vi "Node.Settings.vi"(6 "Action":enum8{"Get", "Set"}(ring), 8 "error in (no error)":errorcluster, 10 "Node.Settings":T1 {"Name" format="%.0x"}, 11 "Item Ref in":T2 format="%.0x") -> (0 "error out":errorcluster, 2 "Node.Settings":T1 {"Name" format="%.0x"}, 3 "Item Ref out":T2 format="%.0x")   [LabVIEW 2023, in "J1939 Addon Shared.lvlib"]
uses:
  J1939 Addon Shared.lvlib
  <vilib>/NI VeriStand/Custom Device API/Custom Device Item Ref.ctl
  Types/Monitor Settings.ctl
  Constants.vi
  <vilib>/NI/NI VeriStand Advanced SysDef API/_SubVIs/SysDef.Property.Set.U32.vi
  <vilib>/NI/NI VeriStand Advanced SysDef API/_SubVIs/SysDef.Property.Set.String.vi
  <vilib>/NI/NI VeriStand Advanced SysDef API/_SubVIs/SysDef.Property.Set.Boolean.vi
  <vilib>/NI VeriStand/Custom Device API/Get Item Property (U32).vi
  <vilib>/NI VeriStand/Custom Device API/Get Item Property (String).vi
  <vilib>/NI VeriStand/Custom Device API/Get Item Property (Boolean).vi
  <vilib>/NI VeriStand/Custom Device API/Custom Device API.lvlib
  <vilib>/NI/NI VeriStand Advanced SysDef API/SysDef API/Advanced System Definition.lvlib
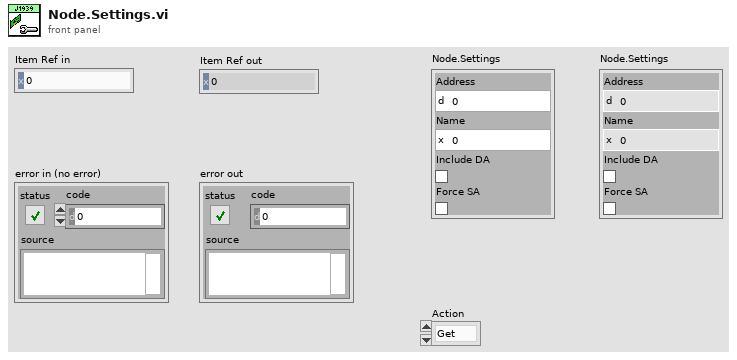
[diagram p1: front panel]
types:
  T1 = typedef "J1939 Addon Shared.lvlib/Monitor Settings.ctl" = cluster{"Address":u8, "Name":u64, "Include DA":bool, "Force SA":bool}
  T2 = typedef "Custom Device API.lvlib/Custom Device Item Ref.ctl" = u64
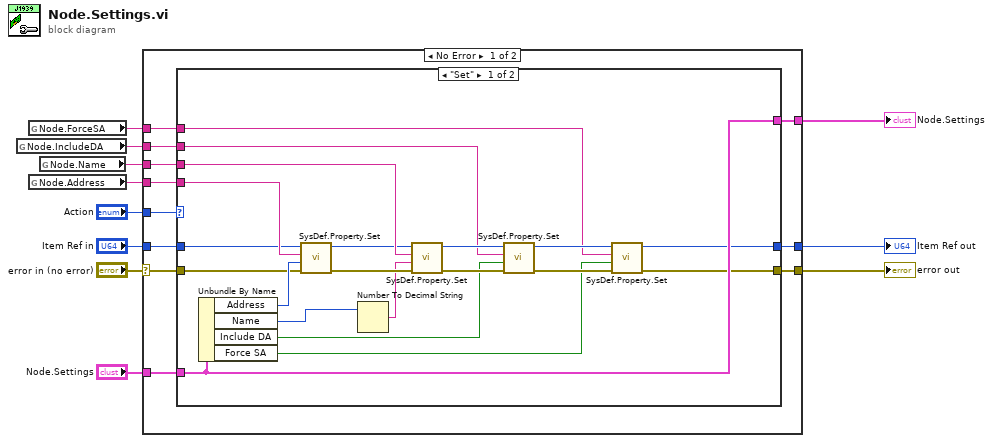
[diagram p0: block diagram]
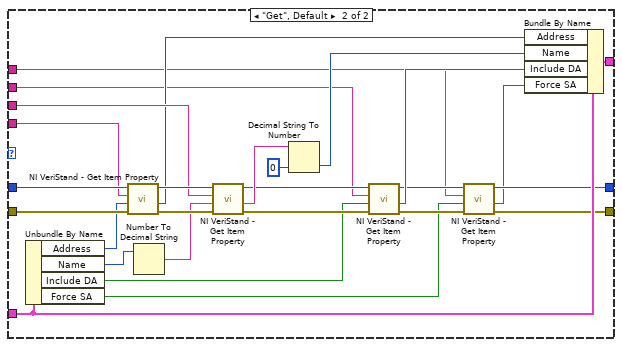
[diagram p2: hidden frame]
diagram:
  n1 = global read "Constants.vi" "Node.IncludeDA"() -> (w2:string)
  n2 = global read "Constants.vi" "Node.ForceSA"() -> (w1:string)
  n3 = global read "Constants.vi" "Node.Address"() -> (w10:string)
  n4 = global read "Constants.vi" "Node.Name"() -> (w6:string)
  n5 = case shown="No Error" "error in (no error)" {
    selector: "error in (no error)" -> [w16 w71]
    tunnel: "Item Ref in" -> [w22 w70]
    tunnel: w10 -> [w21 _]
    tunnel: [w20 w71] -> w9
    tunnel: [w19 w70] -> w8
    tunnel: [w18 _] -> w7
    tunnel: w6 -> [w17 _]
    tunnel: "Node.Settings" -> [w15 _]
    tunnel: "Action" -> [w14 _]
    tunnel: w2 -> [w13 _]
    tunnel: w1 -> [w12 _]
    frame No Error {
      n6 = case shown="\"Set\"" w14 {
        tunnel: w22 -> [w39 w65]
        tunnel: w21 -> [w42 w61]
        tunnel: [w26 w46] -> w20
        tunnel: [w25 w48] -> w19
        tunnel: [w40 w69] -> w18
        tunnel: w17 -> [w41 w60]
        tunnel: w16 -> [w34 w66]
        tunnel: w15 -> [w40 w63]
        tunnel: w13 -> [w29 w52]
        tunnel: w12 -> [w24 w45]
        frame "Set" {
          n7 = Unbundle By Name(w40) -> ("Address"=w36:u8, "Name"=w35:u64, "Include DA"=w30:bool, "Force SA"=w23:bool)
          n8 = call-poly <vilib>:"SysDef.Property.Set.vi"("error in (no error)"=w34, "Value"=w36, "Property Name"=w42, "nodeID"=w39) -> ("error out"=w38:errorcluster, "nodeID out"=w37:u64)  [unwired: 6 in]
          n9 = Number To Decimal String(number=w35) -> (decimal integer string=w33:string)  [unwired: 1 in]
          n10 = call-poly <vilib>:"SysDef.Property.Set.vi"("error in (no error)"=w38, "Value"=w33, "Property Name"=w41, "nodeID"=w37) -> ("error out"=w31:errorcluster, "nodeID out"=w32:u64)  [unwired: 6 in]
          n11 = call-poly <vilib>:"SysDef.Property.Set.vi"("error in (no error)"=w31, "Value"=w30, "Property Name"=w29, "nodeID"=w32) -> ("error out"=w28:errorcluster, "nodeID out"=w27:u64)  [unwired: 6 in]
          n12 = call-poly <vilib>:"SysDef.Property.Set.vi"("error in (no error)"=w28, "Value"=w23, "Property Name"=w24, "nodeID"=w27) -> ("error out"=w26:errorcluster, "nodeID out"=w25:u64)  [unwired: 6 in]
        }
        frame "Get", Default {
          n13 = Unbundle By Name(w63) -> ("Address"=w62:u8, "Name"=w64:u64, "Include DA"=w51:bool, "Force SA"=w44:bool)
          n14 = call-poly <vilib>:"NI VeriStand - Get Item Property.vi"("error in (no error)"=w66, "Default Value"=w62, "Property Name"=w61, "Item Ref in"=w65) -> ("error out"=w68:errorcluster, "Value"=w58:u32, "Item Ref out"=w67:T2)  [unwired: 4 in, 1 out]
          n15 = Number To Decimal String(number=w64) -> (decimal integer string=w59:string)  [unwired: 1 in]
          n16 = call-poly <vilib>:"NI VeriStand - Get Item Property.vi"("error in (no error)"=w68, "Default Value"=w59, "Property Name"=w60, "Item Ref in"=w67) -> ("error out"=w53:errorcluster, "Value"=w57:string, "Item Ref out"=w54:T2)  [unwired: 4 in, 1 out]
          n17 = Decimal String To Number(string=w57, default (0L)=u64 0 ("default (0 I32)")) -> (number=w55:u64)  [unwired: 1 in, 1 out]
          n18 = call-poly <vilib>:"NI VeriStand - Get Item Property.vi"("error in (no error)"=w53, "Default Value"=w51, "Property Name"=w52, "Item Ref in"=w54) -> ("error out"=w47:errorcluster, "Value"=w50:bool, "Item Ref out"=w49:T2)  [unwired: 4 in, 1 out]
          n19 = call-poly <vilib>:"NI VeriStand - Get Item Property.vi"("error in (no error)"=w47, "Default Value"=w44, "Property Name"=w45, "Item Ref in"=w49) -> ("error out"=w46:errorcluster, "Value"=w43:bool, "Item Ref out"=w48:T2)  [unwired: 4 in, 1 out]
          n20 = Bundle By Name(cluster=w63, "Address"=w58, "Name"=w55, "Include DA"=w50, "Force SA"=w43) -> (w69:T1)
        }
      }
    }
    frame Error {
    }
  }
  "Item Ref out" <- w8
  "error out" <- w9
  "Node.Settings" <- w7
